vi "auto match.vi"() -> ()   [LabVIEW 2014]
panel:
  out "# of iterations":dbl
  out "Current Number":dbl
  in  "Number to Match":dbl
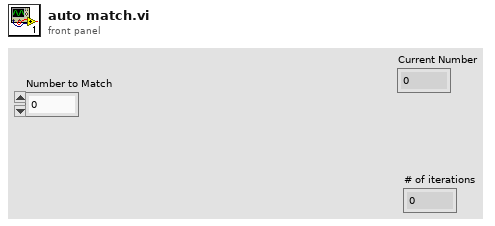
[diagram p1: front panel]
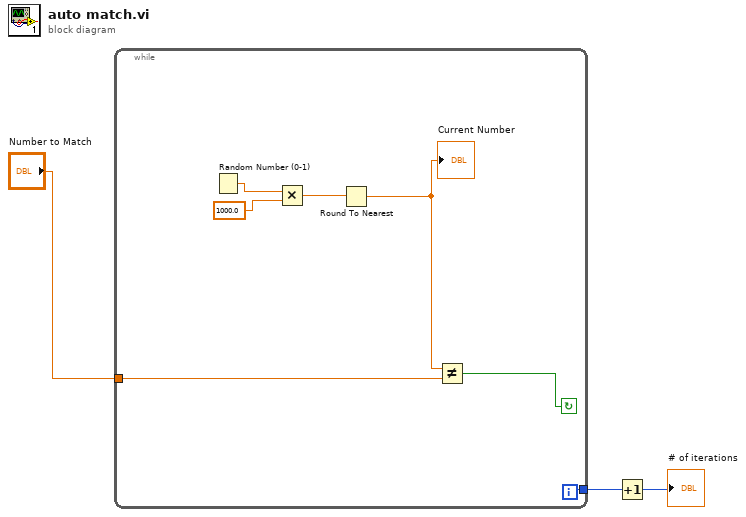
[diagram p0: block diagram]
diagram:
  n1 = while {
    tunnel: "Number to Match" -> [w10]
    tunnel: [w4] -> w1
    i -> [w4]
    stop <- w5 continue-if-true
    n2 = Random Number (0-1)() -> (number: 0 to 1=w8:dbl)
    n3 = Multiply(x=w8, y=1000.0) -> (x*y=w7:dbl)
    n4 = Round To Nearest(number=w7) -> (nearest integer value=w6:dbl)
    "Current Number" <- w6
    n5 = Not Equal?(x=w6, y=w10) -> (x != y?=w5:bool)
  }
  n6 = Increment(x=w1) -> (x+1=→"# of iterations":i32)
